vi "State Estimator complementary.vi"(6 "Configuration":T2={"Accelerometer Bias"={"X (m/s)"=0.0, "Y (m/s)"=0.0, "Z (m/s)"=0.0}, "Gyroscope Bias"={"X (m/s)"=0.0, "Y (m/s)"=0.0, "Z (m/s)"=0.0}, "Steering Motor Gear Ratio"=611.0, "Steering Pully Gear Ratio"=1.0, "Steering Encoder CPR"=500.0, "Steering Motor Max RPM"=4000.0, "Wheelbase (m)"=1.12, "Fork Angle (rad)"=1.3, "Balancing Controller"={"Kp (/s)"=0.0, "Kd (1)"=0.0}, "Max Allowed Steering Angle (rad)"=0.7, "Task Periods"={"Emergency Stop (us)"=0, "IMU (us)"=0, "Steering Motor Encoder (us)"=0, "State Estimator (us)"=0, "Balancing Controller (us)"=0, "GNSS (us)"=0, "Logging (us)"=0, "Drive Motor (us)"=0}, "Drive Motor Gear Ratio"=0.7}, 7 "Ts":dbl, 8 "Measurement In":refnum<data-value>, 11 "Error In":errorcluster) -> (0 "Measurement Out":refnum<data-value>, 3 "Error out":errorcluster)   [LabVIEW 2021]
uses:
  Measurements.ctl
  IMU/IMU Data.ctl
  Steering Motor Encoder/Steering Motor Encoder Data.ctl
  GNSS/GNSS Data.ctl
  Configuration/Configuration.ctl
  State Estimate.ctl
panel:
  out "output cluster":T1
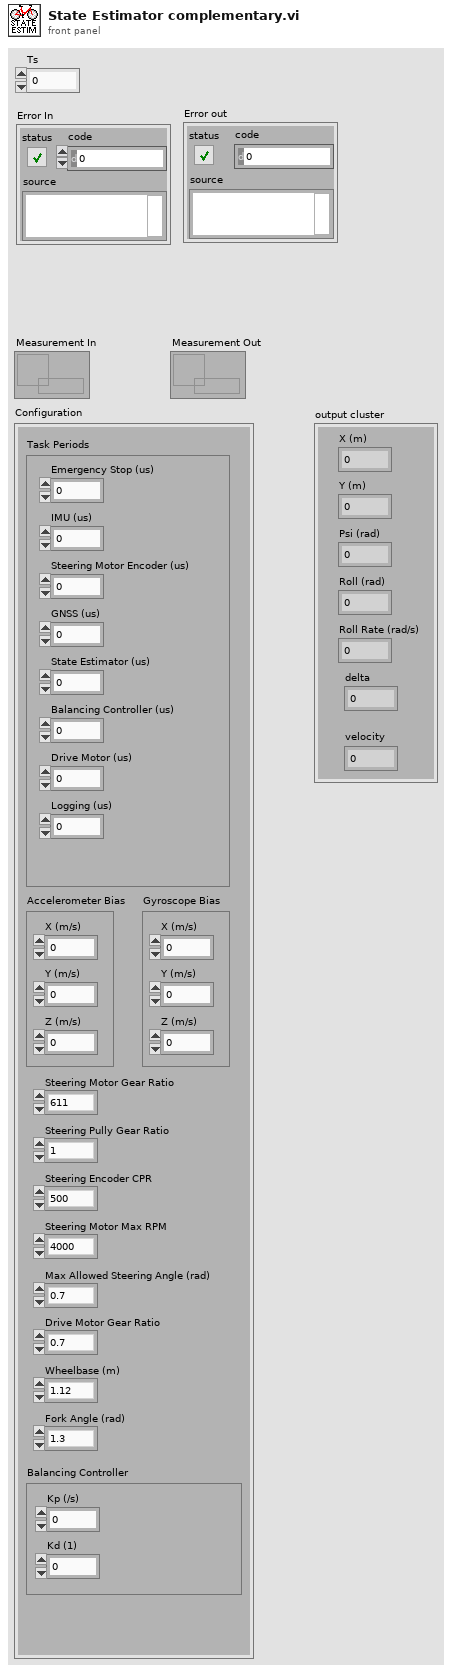
[diagram p1: front panel]
types:
  T1 = typedef "State Estimate.ctl" = cluster{"X (m)":dbl, "Y (m)":dbl, "Psi (rad)":dbl, "Roll (rad)":dbl, "Roll Rate (rad/s)":dbl, "delta":dbl, "velocity":dbl}
  T2 = typedef "Configuration.ctl" = cluster{"Accelerometer Bias":cluster{"X (m/s)":dbl, "Y (m/s)":dbl, "Z (m/s)":dbl}, "Gyroscope Bias":cluster{"X (m/s)":dbl, "Y (m/s)":dbl, "Z (m/s)":dbl}, "Steering Motor Gear Ratio":dbl, "Steering Pully Gear Ratio":dbl, "Steering Encoder CPR":dbl, "Steering Motor Max RPM":dbl, "Wheelbase (m)":dbl, "Fork Angle (rad)":dbl, "Balancing Controller":cluster{"Kp (/s)":dbl, "Kd (1)":dbl}, "Max Allowed Steering Angle (rad)":dbl, "Task Periods":cluster{"Emergency Stop (us)":i64, "IMU (us)":i64, "Steering Motor Encoder (us)":i64, "State Estimator (us)":i64, "Balancing Controller (us)":i64, "GNSS (us)":i64, "Logging (us)":i64, "Drive Motor (us)":i64}, "Drive Motor Gear Ratio":dbl}
  T3 = typedef "Measurements.ctl" = cluster{"IMU Data":T4, "Steering Motor Encoder Data":T5, "GNSS Data":T6}
  T4 = typedef "IMU Data.ctl" = cluster{"Gyroscope":cluster{"X (rad/s)":dbl, "Y (rad/s)":dbl, "Z (rad/s)":dbl}, "Accelerometer":cluster{"X (m/s^2)":dbl, "Y (m/s^2)":dbl, "Z (m/s^2)":dbl}, "Flag IMU":dbl}
  T5 = typedef "Steering Motor Encoder Data.ctl" = cluster{"Encoder Position (counts)":i32, "Steering Angle (rad)":dbl, "Flag Steering Encoder":dbl}
  T6 = typedef "GNSS Data.ctl" = cluster{"Latitude (rad)":dbl, "Longitude (rad)":dbl, "Altitude (m)":dbl, "Speed (m/s)":dbl, "Heading (rad)":dbl, "Fix Quality":i32, "Number of Satellites":i32, "Latitude (deg)":dbl, "Longitude (deg)":dbl, "Flag GNSS":dbl}
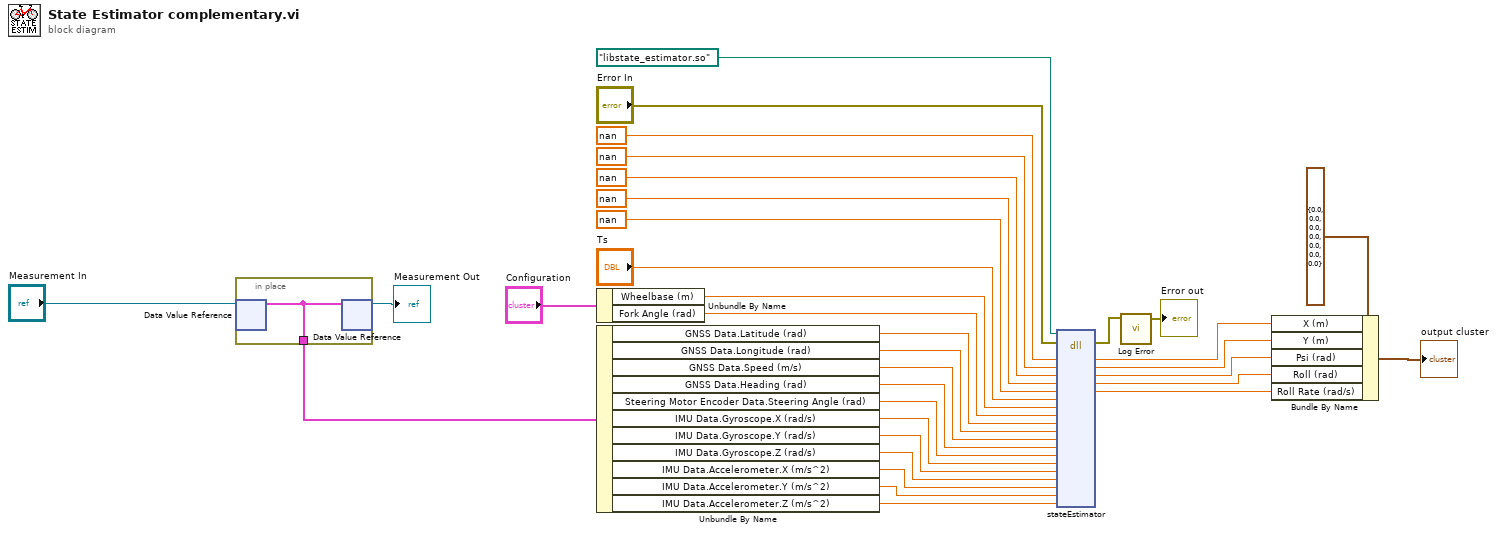
[diagram p0: block diagram]
diagram:
  n1 = in-place {
    in-place-border: [w35] -> w2
    n2 = in-place-dvr #1("Measurement In") -> (w35:T3)  [unwired: 1 out]
    n3 = in-place-dvr #1(w35) -> (→"Measurement Out":refnum<data-value>)  [unwired: 1 out]
  }
  n4 = Unbundle By Name("Configuration") -> ("Wheelbase (m)"=w24:dbl, "Fork Angle (rad)"=w23:dbl)
  n5 = Unbundle By Name(w2) -> ("GNSS Data.Latitude (rad)"=w22:dbl, "GNSS Data.Longitude (rad)"=w21:dbl, "GNSS Data.Speed (m/s)"=w20:dbl, "GNSS Data.Heading (rad)"=w5:dbl, "Steering Motor Encoder Data.Steering Angle (rad)"=w19:dbl, "IMU Data.Gyroscope.X (rad/s)"=w18:dbl, "IMU Data.Gyroscope.Y (rad/s)"=w17:dbl, "IMU Data.Gyroscope.Z (rad/s)"=w16:dbl, "IMU Data.Accelerometer.X (m/s^2)"=w15:dbl, "IMU Data.Accelerometer.Y (m/s^2)"=w14:dbl, "IMU Data.Accelerometer.Z (m/s^2)"=w13:dbl)
  n6 = dll-call lib="?" fn="stateEstimator"(path in=path "libstate_estimator.so", error in="Error In", "X"=nan, "Y"=nan ("X"), "Psi"=nan ("X"), "roll"=nan ("X"), "rollRate"=nan ("X"), "Ts"="Ts", "wheelbase"=w24, "forkAngle"=w23, "latitude"=w22, "longitude"=w21, "speed"=w20, "headingAngle"=w5, "steeringAngle"=w19, "gyroX"=w18, "gyroY"=w17, "gyroZ"=w16, "accX"=w15, "accY"=w14, "accZ"=w13) -> (error out=w3:errorcluster, "X"=w10:dbl, "Y"=w9:dbl, "Psi"=w8:dbl, "roll"=w7:dbl, "rollRate"=w11:dbl)  [unwired: 16 in, 1 out]
  n7 = call "Log Error.vi"("Error In"=w3) -> ("Error Out"=→"Error out":errorcluster)  [unwired: 10 in]
  n8 = Bundle By Name(cluster=T1 {"X (m)"=0.0, "Y (m)"=0.0, "Psi (rad)"=0.0, "Roll (rad)"=0.0, "Roll Rate (rad/s)"=0.0, "delta"=0.0, "velocity"=0.0} ("State Estimate"), "X (m)"=w10, "Y (m)"=w9, "Psi (rad)"=w8, "Roll (rad)"=w7, "Roll Rate (rad/s)"=w11) -> (→"output cluster":T1)
